vi "Combine Offsets.vi"(8 "error in (no error)":errorcluster) -> (0 "error out":errorcluster)   [LabVIEW 2009]
uses:
  Global Data/Transactions/Dataset Type.ctl
  Global Data/Transactions/Dataset Source.ctl
  Global Data/Transactions/Dataset Transaction Id.ctl
  Apps/Yes No Button.ctl
  Data Access Objects/Metadata/DAO Actions.ctl
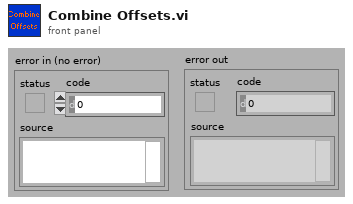
[diagram p1: front panel]
types:
  T1 = typedef "Dataset Transaction Id.ctl" = cluster{"Dataset Source":T2, "Dataset Type":T3, "Hold":T4, "Volts":T4, "Tag":string}
  T2 = typedef "Dataset Source.ctl" = enum16{"LBCB 1", "LBCB 2", "Combined", "External Sensors"}
  T3 = typedef "Dataset Type.ctl" = enum16{"LVDT", "Load Cell", "Actuator Command", "Servo Error", "Displacement Command", "Displacement", "Force"}
  T4 = typedef "Yes No Button.ctl" = bool
  T5 = typedef "DAO Actions.ctl" = enum16{"Init", "Get", "Set"}
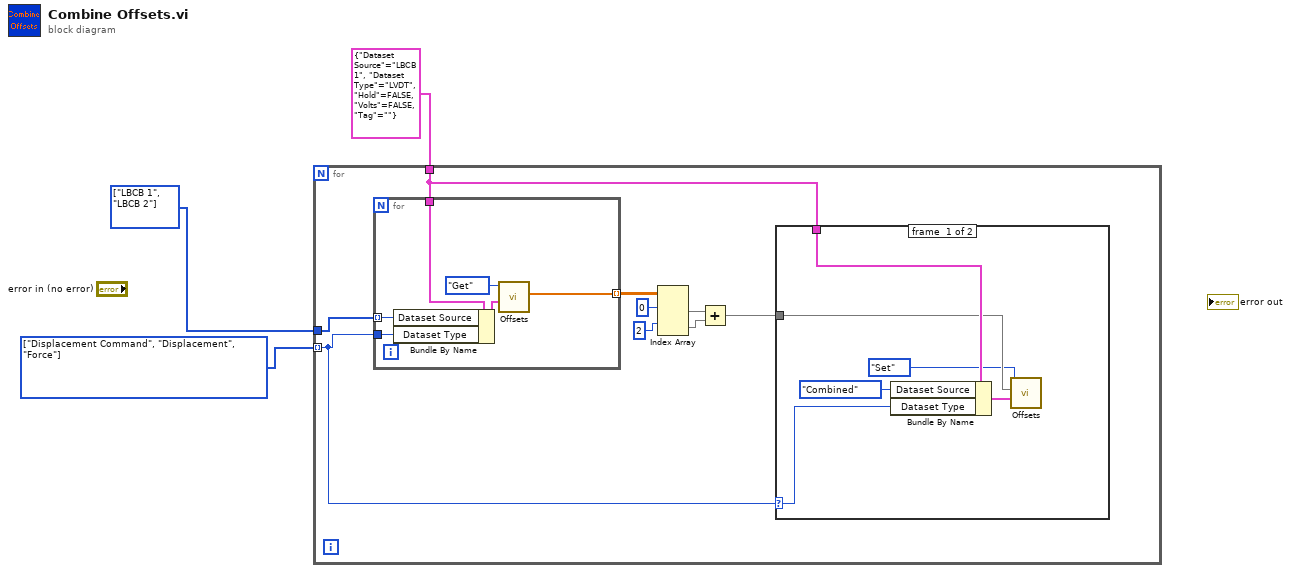
[diagram p0: block diagram]
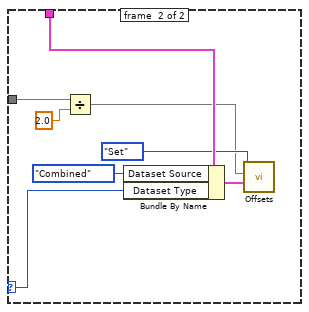
[diagram p2: hidden frame]
diagram:
  w2 = T2[] [enum."LBCB 1", enum."LBCB 2"] items=["LBCB 1", "LBCB 2", "Combined", "External Sensors"]
  w1 = T3[] [enum."Displacement Command", enum."Displacement", enum."Force"] items=["LVDT", "Load Cell", "Actuator Command", "Servo Error", "Displacement Command", "Displacement", "Force"]
  n1 = for {
    tunnel: T1 {"Dataset Source"=enum."LBCB 1", "Dataset Type"=enum."LVDT", "Hold"=FALSE, "Volts"=FALSE, "Tag"=""} ("Dataset Trans Id") -> [w11]
    tunnel: w2 -> [w12]
    tunnel: w1 -> [w9] mode=indexing
    n2 = for {
      tunnel: w11 -> [w31]
      tunnel: w12 -> [w29] mode=indexing
      tunnel: w9 -> [w28]
      tunnel: [w27] -> w10 mode=indexing
      n3 = Bundle By Name(cluster=w31, "Dataset Source"=w29, "Dataset Type"=w28) -> (w30:T1)
      n4 = call "Offsets.vi"("Dataset Trans Id"=w30, "DAO Actions"=DAO_Actions."Get") -> ("Data Out"=w27:dbl[])  [unwired: 7 in, 2 out]
    }
    n5 = Index Array(array=w10, index (row) #1=0 ("index (row)"), index (row) #2=2 ("index (row)")) -> (element #1=w6:dbl[], element #2=w5:dbl[])  [unwired: 2 in]
    n6 = Add(x=w6, y=w5) -> (x+y=w4:dbl[])
    n7 = case shown="\"Displacement Command\", Default" w9 {
      selector: w9 -> [w14 w22]
      tunnel: w11 -> [w18 w26]
      tunnel: w4 -> [w16 w24]
      frame #0 {
        n8 = Bundle By Name(cluster=w18, "Dataset Source"=Dataset_Source."Combined", "Dataset Type"=w14) -> (w17:T1)
        n9 = call "Offsets.vi"("Dataset Trans Id"=w17, "Data In"=w16, "DAO Actions"=DAO_Actions."Set") -> ()  [unwired: 6 in, 3 out]
      }
      frame #1 {
        n10 = Divide(x=w24, y=2.0) -> (x/y=w20:dbl[])
        n11 = Bundle By Name(cluster=w26, "Dataset Source"=Dataset_Source."Combined", "Dataset Type"=w22) -> (w25:T1)
        n12 = call "Offsets.vi"("Dataset Trans Id"=w25, "Data In"=w20, "DAO Actions"=DAO_Actions."Set") -> ()  [unwired: 6 in, 3 out]
      }
    }
  }
